vi "Success.vi"() -> ()   [LabVIEW 2014]
doc: "Tank Drive Example\n\nThis example shows how to implement tank drive and uses two joysticks for input.\n\nThis example expects a USB cable connected from your development PC to the Type B USB Jack (next to the power input) on the roboRIO.\n\nThis example requires the Driver Station to be running with Teleoperated Enabled."
uses:
  <vilib>/Rock Robotics/SystemInterfaces/DIO/FPGA_DIOPWMChannel.ctl
  <vilib>/Rock Robotics/WPI/Joystick/WPI_JoystickDeviceEnum.ctl
  <vilib>/Rock Robotics/WPI/Solenoid/WPI_SolenoidChannel.ctl
  <vilib>/Rock Robotics/WPI/RobotDrive/WPI_RobotDriveOpen2MotorWithTalon.vi
  <vilib>/Rock Robotics/WPI/RobotDrive/WPI_RobotDriveOpen4MotorWithTalon.vi
  <vilib>/Rock Robotics/WPI/Solenoid/WPI_SolenoidOpenSingle.vi
  <vilib>/Rock Robotics/WPI/Joystick/WPI_JoystickGetSetRefNum.vi
  <vilib>/Rock Robotics/WPI/Solenoid/WPI_SolenoidSetEnum.vi
panel:
  in  "stop 2":bool
  in  "stop":bool
  # "Set these inputs before running."
  # "This example requires the Driver Station to be running with Teleoperated Enabled."
  # "PWM cables"
  # "This shows wiring for Talon speed controllers.  The wiring is similar for Victor and Jaguar controllers.  If you change the controller type, you must also select the appropriate instance of the Motor Open VI on the diagram."
  # "Power\nTerminals"
  # "Motor\nTerminals"
  # "+"
  # "+"
  # "M"
  # "B"
  # "Power\nTerminals"
  # "Motor\nTerminals"
  # "+"
  # "+"
  # "M"
  # "B"
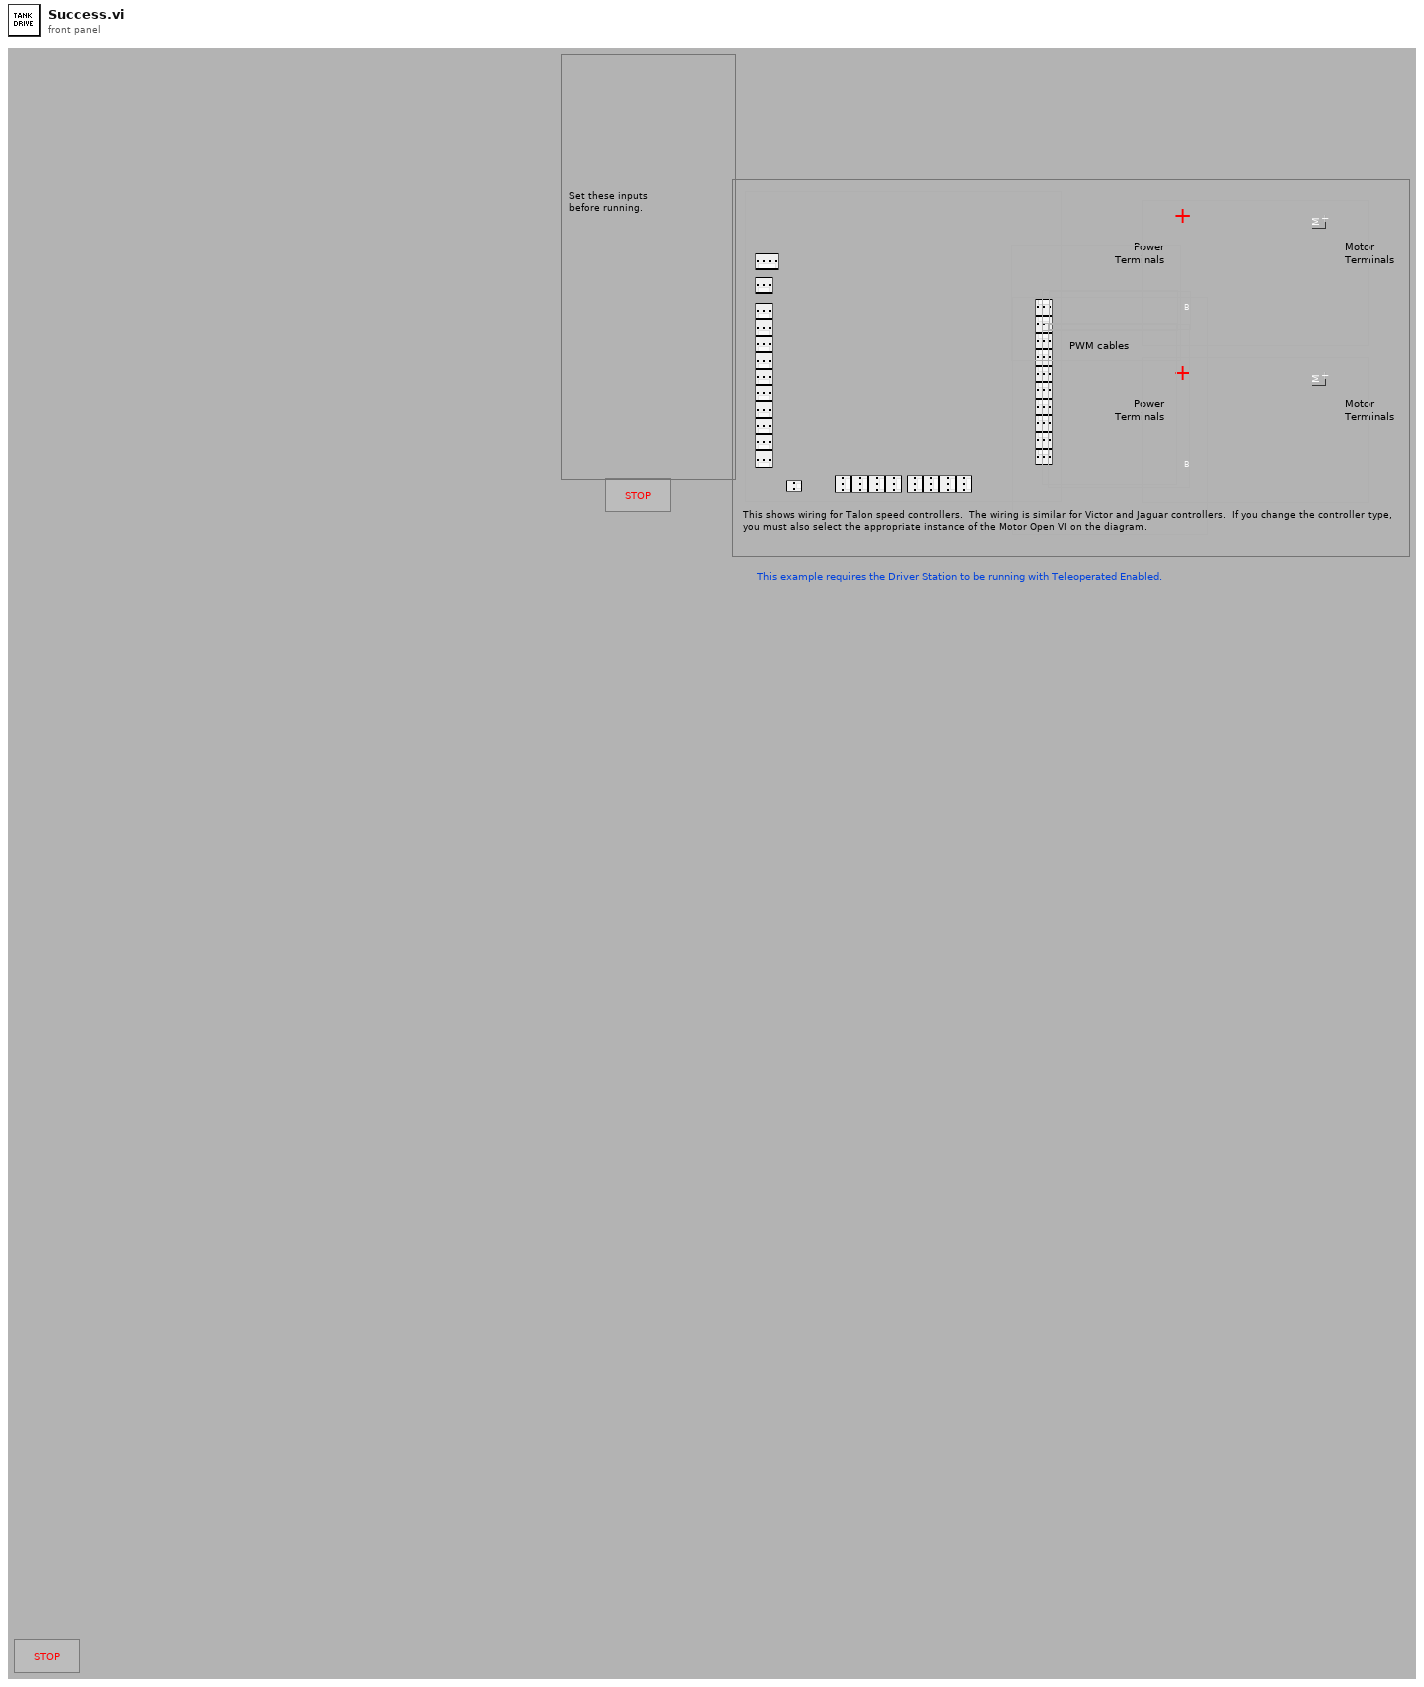
[diagram p1: front panel]
types:
  T1 = typedef "WPI_SolenoidChannel.ctl" = enum8{"Solenoid 0", "Solenoid 1", "Solenoid 2", "Solenoid 3", "Solenoid 4", "Solenoid 5", "Solenoid 6", "Solenoid 7", "Invalid"}
  T2 = typedef "WPI_JoystickDeviceEnum.ctl" = enum16{"USB 0", "USB 1", "USB 2", "USB 3", "USB 4", "USB 5"}
  T3 = typedef "FPGA_DIOPWMChannel.ctl" = enum8{"PWM 0", "PWM 1", "PWM 2", "PWM 3", "PWM 4", "PWM 5", "PWM 6", "PWM 7", "PWM 8", "PWM 9", "PWM MXP 0", "PWM MXP 1", "PWM MXP 2", "PWM MXP 3", "PWM MXP 4", "PWM MXP 5", "PWM MXP 6", "PWM MXP 7", "PWM MXP 8", "PWM MXP 9", "Invalid"}
  T4 = typedef "WPI_JoystickDevRef.ctl" = cluster{"Device":T2}
  T5 = typedef "WPI_SolenoidDevRef.ctl" = cluster{"DevStatus":errorcluster, "Pneumatics Control Module":u8, "Forward Solenoid Channel":T1, "Reverse Solenoid Channel":T1}
  T6 = typedef "WPI_RobotDriveDevRef.ctl" = cluster{"DevStatus":errorcluster, "Motors[]":T7[], "Square Inputs":bool, "Max Output":dbl}
  T7 = typedef "WPI_MotorControlDeviceRef.ctl" = cluster{"DeviceStatus":errorcluster, "Type":T8, "PWM":cluster{"Controller":T9, "PWM Channel":T3, "DeadBand":T10}, "CAN":cluster{"Device Number":u8, "Control Mode":T11, "Semaphore":T12, "Max Vout":dbl, "TalonSRX Control Mode":T13}, "Invert":bool, "TransformRef":T14, "InvTransformRef":T14}
  T8 = typedef "WPI_MotorControlType.ctl" = enum16{"PWM", "CAN", "CANTalonSRX"}
  T9 = typedef "FPGA_TypedefDigitalModule.ctl" = enum16{"Controller 1"}
  T10 = typedef "WPI_PWMDeadband.ctl" = cluster{"Name":string, "maxPositivePwm":i32, "minPositivePwm":i32, "centerPwm":i32, "maxNegativePwm":i32, "minNegativePwm":i32, "angularRange":u16}
  T11 = typedef "WPI_CANJaguar_ControlMode.ctl" = enum8{"Percent VBus", "Current", "Speed", "Position", "Voltage"}
  T12 = typedef "Semaphore RefNum" = refnum<k1>
  T13 = typedef "WPI_CANTalonSRX_APIControlMode.ctl" = enum8{"Percent VBus", "Speed", "Position", "Slave", "Unchanged / Invalid"}
  T14 = typedef "WPI_PWMTransform_ConPane.ctl" = refnum<vi>
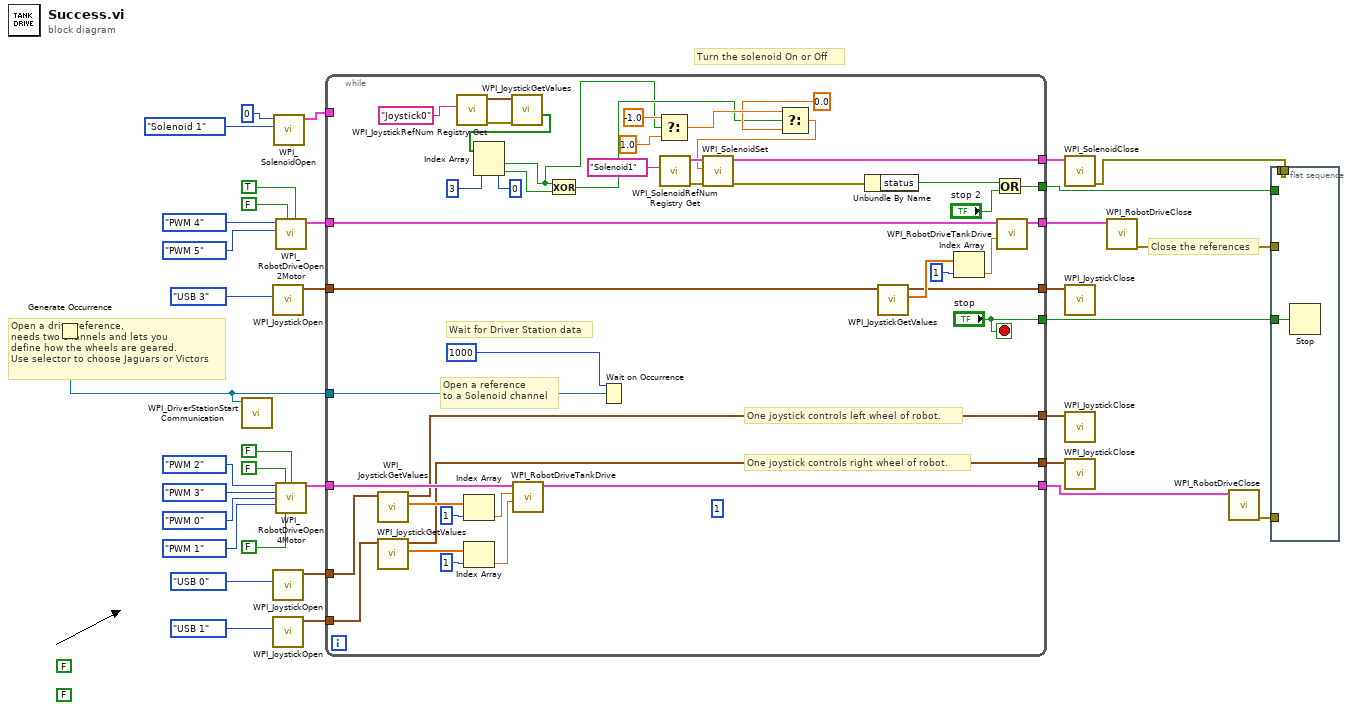
[diagram p0: block diagram]
diagram:
  (unwired) FALSE ("Right Motor Inverted")
  (unwired) FALSE ("Left Motor Inverted")
  # "Turn the solenoid On or Off"
  # "Close the references"
  # "Open a drive reference,\nneeds two channels and lets you\ndefine how the wheels are geared.\nUse selector to choose Jaguars or Victors"
  n1 = Generate Occurrence() -> (w33:refnum<k4>)
  n2 = call <vilib>:"WPI_DriverStationStart Communication.vi"("occurrence"=w33) -> ()  [unwired: 1 in, 10 out]
  n3 = call <vilib>:"WPI_JoystickOpen.vi"("JoystickDevice"=WPI_JoystickDeviceEnum."USB 3") -> ("JoystickDevRef"=w10:T4)  [unwired: 10 out]
  n4 = call <vilib>:"WPI_JoystickOpen.vi"("JoystickDevice"=WPI_JoystickDeviceEnum."USB 0" ("LeftStick")) -> ("JoystickDevRef"=w29:T4)  [unwired: 10 out]
  n5 = call <vilib>:"WPI_JoystickOpen.vi"("JoystickDevice"=WPI_JoystickDeviceEnum."USB 1" ("RightStick")) -> ("JoystickDevRef"=w30:T4)  [unwired: 10 out]
  n6 = call-poly <vilib>:"WPI_SolenoidOpen.vi"("Solenoid Channel"=WPI_SolenoidChannel."Solenoid 1", "Pneumatics Control Module (0)"=u8 0) -> ("SolenoidDevRef"=w2:T5)  [unwired: 8 in, 1 out]
  n7 = call-poly <vilib>:"WPI_RobotDriveOpen2Motor.vi"("Right Motor Inverted"=TRUE, "Left Motor Inverted"=FALSE, "Right Motor"=FPGA_DIOPWMChannel."PWM 5", "Left Motor"=FPGA_DIOPWMChannel."PWM 4") -> ("RobotDriveDevRef"=w8:T6)  [unwired: 6 in, 1 out]
  n8 = call-poly <vilib>:"WPI_RobotDriveOpen4Motor.vi"("Rear Left Motor"=FPGA_DIOPWMChannel."PWM 2" ("Left Motor (PWM channel)"), "Rear Left Motor Inverted"=FALSE, "Rear Right Motor Inverted"=FALSE, "Rear Right Motor"=FPGA_DIOPWMChannel."PWM 3" ("Right Motor (PWM channel)"), "Front Left Motor"=FPGA_DIOPWMChannel."PWM 0", "Front Right Motor"=FPGA_DIOPWMChannel."PWM 1", "Front Left Motor Inverted"=FALSE) -> ("RobotDriveDevRef"=w22:T6)  [unwired: 7 in, 1 out]
  n9 = while {
    tunnel: w22 -> [w73]
    tunnel: [w74] -> w34
    tunnel: w33 -> [w78]
    tunnel: ["stop"] -> w26
    tunnel: w30 -> [w76]
    tunnel: w29 -> [w75]
    tunnel: [w71] -> w28
    tunnel: [w70] -> w27
    tunnel: [w61] -> w16
    tunnel: [w59] -> w15
    tunnel: [w57] -> w11
    tunnel: w10 -> [w35]
    tunnel: w8 -> [w56]
    tunnel: [w55] -> w7
    tunnel: w2 -> [_]
    stop <- "stop" stop-if-true
    (unwired) 1 ("index")
    # "Open a reference \nto a Solenoid channel"
    # "Wait for Driver Station data"
    # "One joystick controls right wheel of robot."
    # "One joystick controls left wheel of robot."
    n10 = call <vilib>:"WPI_JoystickGetValues.vi"("JoystickDevRef"=w75) -> ("Axes"=w72:dbl[], "JoystickDevRef"=w71:T4)  [unwired: 6 in, 3 out]
    n11 = call <vilib>:"WPI_JoystickGetValues.vi"("JoystickDevRef"=w76) -> ("Axes"=w67:dbl[], "JoystickDevRef"=w70:T4)  [unwired: 6 in, 3 out]
    n12 = call <vilib>:"WPI_JoystickRefNum Registry Get.vi"("refnum name"="Joystick0") -> ("error out"=w38:errorcluster, "JoystickDevRef"=w37:T4)  [unwired: 9 in]
    n13 = Index Array(array=w72, index=1) -> (element=w66:dbl)
    n14 = Index Array(array=w67, index=1) -> (element=w65:dbl)
    n15 = call <vilib>:"WPI_JoystickGetValues.vi"("error in (no error)"=w38, "JoystickDevRef"=w37) -> ("Buttons"=w36:bool[])  [unwired: 5 in, 4 out]
    n16 = Index Array(array=w36, index #1=0 ("index"), index #2=3 ("index")) -> (element #1=w40:bool, element #2=w47:bool)
    n17 = call <vilib>:"WPI_RobotDriveTankDrive.vi"("Right axis value"=w65, "Left axis value"=w66, "RobotDriveDevRef"=w73) -> ("RobotDriveDevRef"=w74:T6)  [unwired: 1 in, 7 out]
    n18 = Exclusive Or(1:w47, 2:w40) -> (0:w41:bool)
    n19 = Wait on Occurrence(2:w78, 3:1000 ("ms timeout (-1)")) -> ()  [unwired: 2 out]
    n20 = Select(t=-1.0, s=w40, f=1.0) -> (s? t:f=w44:dbl)
    n21 = call <vilib>:"WPI_SolenoidRefNum Registry Get.vi"("refnum name"="Solenoid1") -> ("error out"=w51:errorcluster, "SolenoidDevRef"=w52:T5)  [unwired: 9 in]
    n22 = Select(t=w44, s=w41, f=0.0) -> (s? t:f=w42:dbl)
    n23 = call-poly <vilib>:"WPI_SolenoidSet.vi"("error in (no error)"=w51, "Value"=w42, "SolenoidDevRef"=w52) -> ("error out"=w64:errorcluster, "SolenoidDevRef"=w61:T5)  [unwired: 7 out]
    n24 = Unbundle By Name(w64) -> ("status"=w63:bool)
    n25 = call <vilib>:"WPI_JoystickGetValues.vi"("JoystickDevRef"=w35) -> ("Axes"=w58:dbl[], "JoystickDevRef"=w57:T4)  [unwired: 6 in, 3 out]
    n26 = Index Array(array=w58, index=1) -> (element=w53:dbl)
    n27 = Or(x=w63, y="stop 2") -> (x .or. y?=w59:bool)
    n28 = call <vilib>:"WPI_RobotDriveTankDrive.vi"("Right axis value"=w53, "RobotDriveDevRef"=w56) -> ("RobotDriveDevRef"=w55:T6)  [unwired: 7 in, 2 out]
  }
  n29 = call <vilib>:"WPI_SolenoidClose.vi"("SolenoidDevRef"=w16) -> ("error out"=w1:errorcluster)  [unwired: 10 in]
  n30 = call <vilib>:"WPI_JoystickClose.vi"("JoystickDevRef"=w11) -> ()  [unwired: 11 in]
  n31 = call <vilib>:"WPI_JoystickClose.vi"("JoystickDevRef"=w28) -> ()  [unwired: 11 out]
  n32 = call <vilib>:"WPI_JoystickClose.vi"("JoystickDevRef"=w27) -> ()  [unwired: 11 out]
  n33 = call <vilib>:"WPI_RobotDriveClose.vi"("RobotDriveDevRef"=w7) -> ("error out"=w9:errorcluster)  [unwired: 10 in]
  n34 = call <vilib>:"WPI_RobotDriveClose.vi"("RobotDriveDevRef"=w34) -> ("error out"=w25:errorcluster)  [unwired: 1 in, 9 out]
  n35 = flat-sequence {
    tunnel: w26 -> [w80]
    tunnel: w25 -> [_]
    tunnel: w15 -> [_]
    tunnel: w9 -> [_]
    tunnel: [w79] -> _
    tunnel: w1 -> [w79]
    frame #0 {
      n36 = Stop(stop? (T)=w80) -> ()
    }
  }
